vi "button commands.vi"(6 "Configuration":T1, 8 "Motion":T2, 9 "Y Steps":dbl, 10 "mapped gp buttons":T3, 11 "X Steps":dbl) -> (0 "Y distance":dbl, 1 "Choose Button":bool, 3 "X distance":dbl)   [LabVIEW 2012]
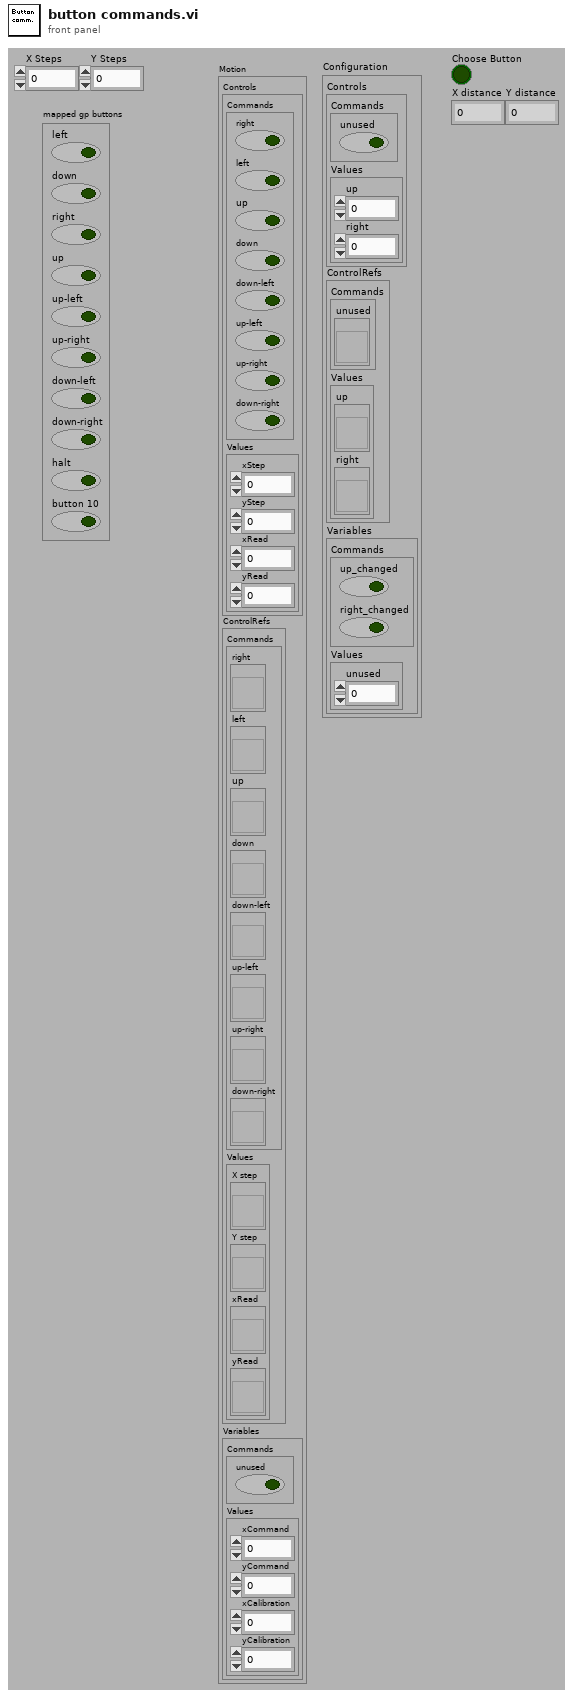
[diagram p1: front panel]
types:
  T1 = cluster{"Controls":cluster{"Commands":cluster{"unused":bool}, "Values":cluster{"up":u16, "right":u16}}, "ControlRefs":cluster{"Commands":cluster{"unused":refnum<vi>}, "Values":cluster{"up":refnum<vi>, "right":refnum<vi>}}, "Variables":cluster{"Commands":cluster{"up_changed":bool, "right_changed":bool}, "Values":cluster{"unused":i32}}}
  T2 = cluster{"Controls":cluster{"Commands":cluster{"right":bool, "left":bool, "up":bool, "down":bool, "down-left":bool, "up-left":bool, "up-right":bool, "down-right":bool}, "Values":cluster{"xStep":dbl, "yStep":dbl, "xRead":dbl, "yRead":dbl}}, "ControlRefs":cluster{"Commands":cluster{"right":refnum<vi>, "left":refnum<vi>, "up":refnum<vi>, "down":refnum<vi>, "down-left":refnum<vi>, "up-left":refnum<vi>, "up-right":refnum<vi>, "down-right":refnum<vi>}, "Values":cluster{"X step":refnum<vi>, "Y step":refnum<vi>, "xRead":refnum<vi>, "yRead":refnum<vi>}}, "Variables":cluster{"Commands":cluster{"unused":bool}, "Values":cluster{"xCommand":dbl, "yCommand":dbl, "xCalibration":dbl, "yCalibration":dbl}}}
  T3 = cluster{"left":bool, "down":bool, "right":bool, "up":bool, "up-left":bool, "up-right":bool, "down-left":bool, "down-right":bool, "halt":bool, "button 10":bool}
  T4 = cluster{"xf":bool, "xr":bool, "yf":bool, "yr":bool, "yr xr":bool, "yf xr":bool, "yf xf":bool, "yr xf":bool}
  T5 = cluster{"up":bool, "down":bool, "left":bool, "right":bool}
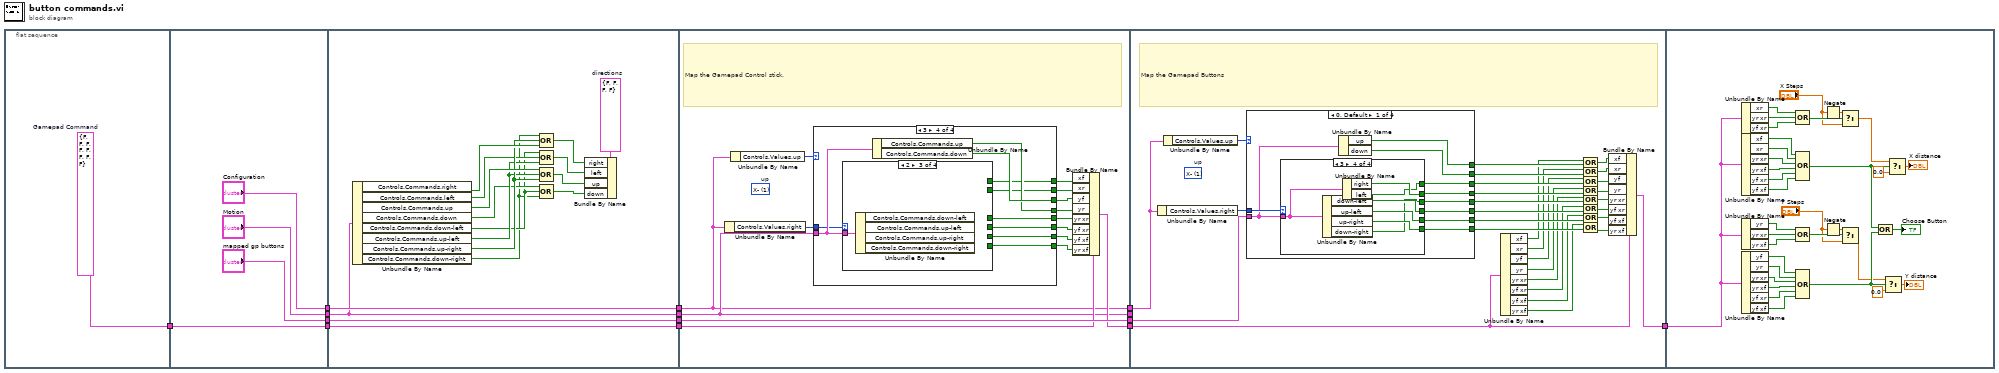
[diagram p0: block diagram]
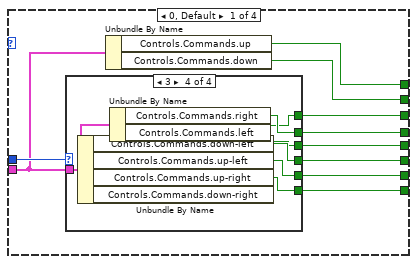
[diagram p2: hidden frame]
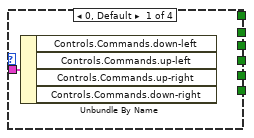
[diagram p3: hidden frame]
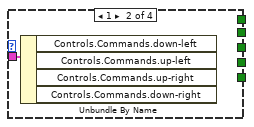
[diagram p4: hidden frame]
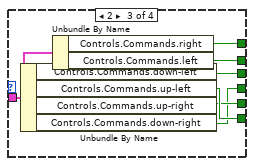
[diagram p5: hidden frame]
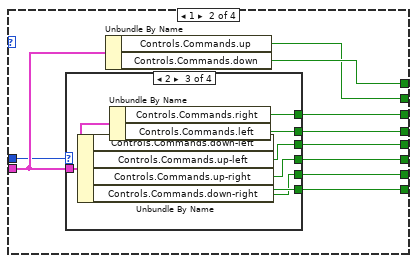
[diagram p6: hidden frame]
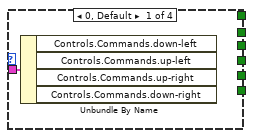
[diagram p7: hidden frame]
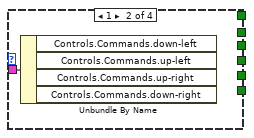
[diagram p8: hidden frame]
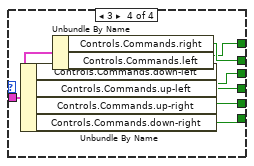
[diagram p9: hidden frame]
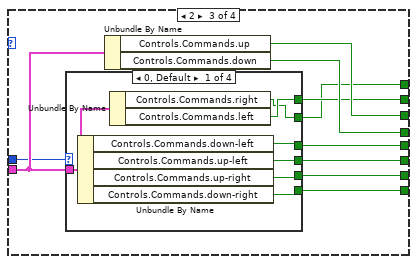
[diagram p10: hidden frame]
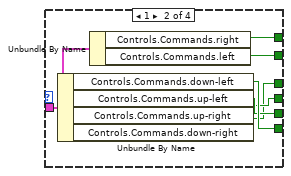
[diagram p11: hidden frame]
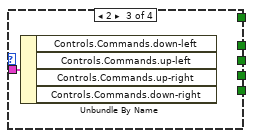
[diagram p12: hidden frame]
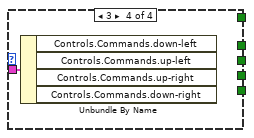
[diagram p13: hidden frame]
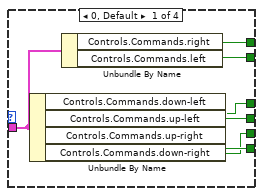
[diagram p14: hidden frame]
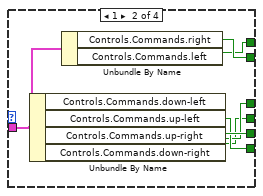
[diagram p15: hidden frame]
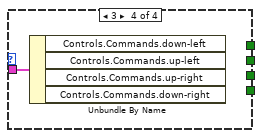
[diagram p16: hidden frame]
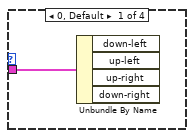
[diagram p17: hidden frame]
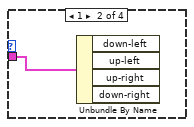
[diagram p18: hidden frame]
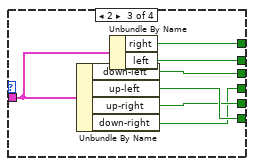
[diagram p19: hidden frame]
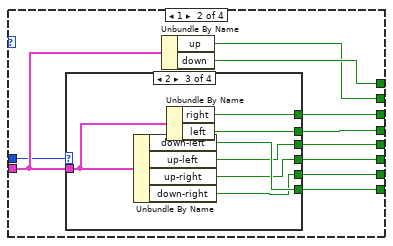
[diagram p20: hidden frame]
diagram:
  n1 = flat-sequence {
    tunnel: [w15] -> w10
    tunnel: ["mapped gp buttons"] -> w9
    tunnel: [w17] -> w8
    tunnel: ["Motion"] -> w7
    tunnel: w10 -> [w17]
    tunnel: ["Configuration"] -> w6
    tunnel: w9 -> [w36]
    tunnel: [w36] -> w5
    tunnel: w8 -> [w35]
    tunnel: [w35] -> w4
    tunnel: w7 -> [w33]
    tunnel: [w33] -> w3
    tunnel: w6 -> [w34]
    tunnel: [w34] -> w2
    tunnel: [w51] -> w13
    tunnel: [w49] -> w12
    tunnel: [w46] -> w11
    tunnel: w2 -> [w37]
    tunnel: w3 -> [w46]
    tunnel: w4 -> [w50]
    tunnel: w5 -> [w51]
    tunnel: [w37] -> w1
    tunnel: w13 -> [w180]
    tunnel: w12 -> [w164]
    tunnel: [w181] -> w14
    tunnel: w11 -> [_]
    tunnel: w1 -> [w182]
    tunnel: w14 -> [w290]
    frame #0 {
      w15 = T4 {"xf"=FALSE, "xr"=FALSE, "yf"=FALSE, "yr"=FALSE, "yr xr"=FALSE, "yf xr"=FALSE, "yf xf"=FALSE, "yr xf"=FALSE}  # Gamepad Command
    }
    frame #1 {
    }
    frame #2 {
      w32 = T5 {"up"=FALSE, "down"=FALSE, "left"=FALSE, "right"=FALSE}  # directions
      n2 = Unbundle By Name(w33) -> ("Controls.Commands.right"=w30:bool, "Controls.Commands.left"=w28:bool, "Controls.Commands.up"=w31:bool, "Controls.Commands.down"=w26:bool, "Controls.Commands.down-left"=w25:bool, "Controls.Commands.up-left"=w27:bool, "Controls.Commands.up-right"=w29:bool, "Controls.Commands.down-right"=w24:bool)
      n3 = Compound Arithmetic op=OR(w24, w29, w30) -> (w23:bool)
      n4 = Compound Arithmetic op=OR(w25, w28, w27) -> (w22:bool)
      n5 = Compound Arithmetic op=OR(w31, w27, w29) -> (w21:bool)
      n6 = Compound Arithmetic op=OR(w26, w25, w24) -> (w20:bool)
      n7 = Bundle By Name(cluster=w32, "right"=w23, "left"=w22, "up"=w21, "down"=w20) -> ()  [unwired: 1 out]
    }
    frame #3 {
      (unwired) u16 1 items=["X+", "X-", "Y+", "Y-"]  # up
      # "Map the Gamepad Control stick."
      n8 = Unbundle By Name(w37) -> ("Controls.Values.right"=w45:u16)
      n9 = Unbundle By Name(w37) -> ("Controls.Values.up"=w48:u16)
      n10 = case shown="3" w48 {
        tunnel: [w61 w81 w104 w130] -> w47
        tunnel: w46 -> [w54 w87 w113 w139]
        tunnel: w45 -> [w60 w86 w112 w138]
        tunnel: [w59 w80 w105 w131] -> w44
        tunnel: [w58 w85 w111 w137] -> w43
        tunnel: [w57 w84 w110 w136] -> w42
        tunnel: [w56 w83 w109 w135] -> w41
        tunnel: [w55 w82 w108 w134] -> w40
        tunnel: [w53 w78 w107 w133] -> w39
        tunnel: [w52 w79 w106 w132] -> w38
        frame 0, Default {
          n11 = case shown="3" w60 {
            tunnel: w54 -> [w62 w63 w66 w73]
            tunnel: [_ _ w70 w74] -> w58
            tunnel: [_ _ w69 w75] -> w57
            tunnel: [_ _ w68 w76] -> w56
            tunnel: [_ _ w67 w77] -> w55
            tunnel: [_ _ w65 w71] -> w53
            tunnel: [_ _ w64 w72] -> w52
            frame 0, Default {
              n12 = Unbundle By Name(w62) -> ()  [unwired: 4 out]
            }
            frame 1 {
              n13 = Unbundle By Name(w63) -> ()  [unwired: 4 out]
            }
            frame 2 {
              n14 = Unbundle By Name(w66) -> ("Controls.Commands.down-left"=w70:bool, "Controls.Commands.up-left"=w69:bool, "Controls.Commands.up-right"=w68:bool, "Controls.Commands.down-right"=w67:bool)
              n15 = Unbundle By Name(w66) -> ("Controls.Commands.right"=w65:bool, "Controls.Commands.left"=w64:bool)
            }
            frame 3 {
              n16 = Unbundle By Name(w73) -> ("Controls.Commands.down-left"=w77:bool, "Controls.Commands.up-left"=w76:bool, "Controls.Commands.up-right"=w75:bool, "Controls.Commands.down-right"=w74:bool)
              n17 = Unbundle By Name(w73) -> ("Controls.Commands.right"=w72:bool, "Controls.Commands.left"=w71:bool)
            }
          }
          n18 = Unbundle By Name(w54) -> ("Controls.Commands.up"=w61:bool, "Controls.Commands.down"=w59:bool)
        }
        frame 1 {
          n19 = case shown="2" w86 {
            tunnel: w87 -> [w88 w89 w92 w99]
            tunnel: [_ _ w95 w101] -> w85
            tunnel: [_ _ w96 w100] -> w84
            tunnel: [_ _ w93 w103] -> w83
            tunnel: [_ _ w94 w102] -> w82
            tunnel: [_ _ w90 w98] -> w79
            tunnel: [_ _ w91 w97] -> w78
            frame 0, Default {
              n20 = Unbundle By Name(w88) -> ()  [unwired: 4 out]
            }
            frame 1 {
              n21 = Unbundle By Name(w89) -> ()  [unwired: 4 out]
            }
            frame 2 {
              n22 = Unbundle By Name(w92) -> ("Controls.Commands.down-left"=w96:bool, "Controls.Commands.up-left"=w95:bool, "Controls.Commands.up-right"=w94:bool, "Controls.Commands.down-right"=w93:bool)
              n23 = Unbundle By Name(w92) -> ("Controls.Commands.right"=w91:bool, "Controls.Commands.left"=w90:bool)
            }
            frame 3 {
              n24 = Unbundle By Name(w99) -> ("Controls.Commands.down-left"=w103:bool, "Controls.Commands.up-left"=w102:bool, "Controls.Commands.up-right"=w101:bool, "Controls.Commands.down-right"=w100:bool)
              n25 = Unbundle By Name(w99) -> ("Controls.Commands.right"=w98:bool, "Controls.Commands.left"=w97:bool)
            }
          }
          n26 = Unbundle By Name(w87) -> ("Controls.Commands.up"=w80:bool, "Controls.Commands.down"=w81:bool)
        }
        frame 2 {
          n27 = case shown="0, Default" w112 {
            tunnel: w113 -> [w116 w123 w128 w129]
            tunnel: [w120 w124 _ _] -> w111
            tunnel: [w117 w127 _ _] -> w110
            tunnel: [w118 w126 _ _] -> w109
            tunnel: [w119 w125 _ _] -> w108
            tunnel: [w115 w122 _ _] -> w105
            tunnel: [w114 w121 _ _] -> w104
            frame 0, Default {
              n28 = Unbundle By Name(w116) -> ("Controls.Commands.down-left"=w120:bool, "Controls.Commands.up-left"=w119:bool, "Controls.Commands.up-right"=w118:bool, "Controls.Commands.down-right"=w117:bool)
              n29 = Unbundle By Name(w116) -> ("Controls.Commands.right"=w114:bool, "Controls.Commands.left"=w115:bool)
            }
            frame 1 {
              n30 = Unbundle By Name(w123) -> ("Controls.Commands.down-left"=w127:bool, "Controls.Commands.up-left"=w126:bool, "Controls.Commands.up-right"=w125:bool, "Controls.Commands.down-right"=w124:bool)
              n31 = Unbundle By Name(w123) -> ("Controls.Commands.right"=w122:bool, "Controls.Commands.left"=w121:bool)
            }
            frame 2 {
              n32 = Unbundle By Name(w128) -> ()  [unwired: 4 out]
            }
            frame 3 {
              n33 = Unbundle By Name(w129) -> ()  [unwired: 4 out]
            }
          }
          n34 = Unbundle By Name(w113) -> ("Controls.Commands.up"=w107:bool, "Controls.Commands.down"=w106:bool)
        }
        frame 3 {
          n35 = case shown="2" w138 {
            tunnel: w139 -> [w142 w149 w154 w155]
            tunnel: [w145 w151 _ _] -> w137
            tunnel: [w144 w152 _ _] -> w136
            tunnel: [w143 w153 _ _] -> w135
            tunnel: [w146 w150 _ _] -> w134
            tunnel: [w140 w148 _ _] -> w131
            tunnel: [w141 w147 _ _] -> w130
            frame 0, Default {
              n36 = Unbundle By Name(w142) -> ("Controls.Commands.down-left"=w146:bool, "Controls.Commands.up-left"=w145:bool, "Controls.Commands.up-right"=w144:bool, "Controls.Commands.down-right"=w143:bool)
              n37 = Unbundle By Name(w142) -> ("Controls.Commands.right"=w141:bool, "Controls.Commands.left"=w140:bool)
            }
            frame 1 {
              n38 = Unbundle By Name(w149) -> ("Controls.Commands.down-left"=w153:bool, "Controls.Commands.up-left"=w152:bool, "Controls.Commands.up-right"=w151:bool, "Controls.Commands.down-right"=w150:bool)
              n39 = Unbundle By Name(w149) -> ("Controls.Commands.right"=w148:bool, "Controls.Commands.left"=w147:bool)
            }
            frame 2 {
              n40 = Unbundle By Name(w154) -> ()  [unwired: 4 out]
            }
            frame 3 {
              n41 = Unbundle By Name(w155) -> ()  [unwired: 4 out]
            }
          }
          n42 = Unbundle By Name(w139) -> ("Controls.Commands.up"=w132:bool, "Controls.Commands.down"=w133:bool)
        }
      }
      n43 = Bundle By Name(cluster=w50, "xf"=w47, "xr"=w44, "yf"=w39, "yr"=w38, "yr xr"=w43, "yf xr"=w40, "yf xf"=w41, "yr xf"=w42) -> (w49:T4)
    }
    frame #4 {
      (unwired) u16 1 items=["X+", "X-", "Y+", "Y-"]  # up
      # "Map the Gamepad Buttons"
      n44 = Unbundle By Name(w182) -> ("Controls.Values.right"=w185:u16)
      n45 = Unbundle By Name(w182) -> ("Controls.Values.up"=w183:u16)
      n46 = case shown="0, Default" w183 {
        tunnel: [w195 w215 w238 w264] -> w184
        tunnel: w180 -> [w188 w221 w247 w273]
        tunnel: w185 -> [w194 w220 w246 w272]
        tunnel: [w193 w214 w239 w265] -> w178
        tunnel: [w192 w219 w245 w271] -> w175
        tunnel: [w191 w218 w244 w270] -> w172
        tunnel: [w190 w217 w243 w269] -> w173
        tunnel: [w189 w216 w242 w268] -> w174
        tunnel: [w187 w212 w241 w267] -> w177
        tunnel: [w186 w213 w240 w266] -> w176
        frame 0, Default {
          n47 = case shown="3" w194 {
            tunnel: w188 -> [w196 w197 w200 w207]
            tunnel: [_ _ w204 w208] -> w192
            tunnel: [_ _ w203 w209] -> w191
            tunnel: [_ _ w202 w210] -> w190
            tunnel: [_ _ w201 w211] -> w189
            tunnel: [_ _ w199 w205] -> w187
            tunnel: [_ _ w198 w206] -> w186
            frame 0, Default {
              n48 = Unbundle By Name(w196) -> ()  [unwired: 4 out]
            }
            frame 1 {
              n49 = Unbundle By Name(w197) -> ()  [unwired: 4 out]
            }
            frame 2 {
              n50 = Unbundle By Name(w200) -> ("down-left"=w204:bool, "up-left"=w203:bool, "up-right"=w202:bool, "down-right"=w201:bool)
              n51 = Unbundle By Name(w200) -> ("right"=w199:bool, "left"=w198:bool)
            }
            frame 3 {
              n52 = Unbundle By Name(w207) -> ("down-left"=w211:bool, "up-left"=w210:bool, "up-right"=w209:bool, "down-right"=w208:bool)
              n53 = Unbundle By Name(w207) -> ("right"=w206:bool, "left"=w205:bool)
            }
          }
          n54 = Unbundle By Name(w188) -> ("up"=w195:bool, "down"=w193:bool)
        }
        frame 1 {
          n55 = case shown="2" w220 {
            tunnel: w221 -> [w222 w223 w226 w233]
            tunnel: [_ _ w229 w235] -> w219
            tunnel: [_ _ w230 w234] -> w218
            tunnel: [_ _ w227 w237] -> w217
            tunnel: [_ _ w228 w236] -> w216
            tunnel: [_ _ w224 w232] -> w213
            tunnel: [_ _ w225 w231] -> w212
            frame 0, Default {
              n56 = Unbundle By Name(w222) -> ()  [unwired: 4 out]
            }
            frame 1 {
              n57 = Unbundle By Name(w223) -> ()  [unwired: 4 out]
            }
            frame 2 {
              n58 = Unbundle By Name(w226) -> ("down-left"=w230:bool, "up-left"=w229:bool, "up-right"=w228:bool, "down-right"=w227:bool)
              n59 = Unbundle By Name(w226) -> ("right"=w225:bool, "left"=w224:bool)
            }
            frame 3 {
              n60 = Unbundle By Name(w233) -> ("down-left"=w237:bool, "up-left"=w236:bool, "up-right"=w235:bool, "down-right"=w234:bool)
              n61 = Unbundle By Name(w233) -> ("right"=w232:bool, "left"=w231:bool)
            }
          }
          n62 = Unbundle By Name(w221) -> ("up"=w214:bool, "down"=w215:bool)
        }
        frame 2 {
          n63 = case shown="0, Default" w246 {
            tunnel: w247 -> [w250 w257 w262 w263]
            tunnel: [w254 w258 _ _] -> w245
            tunnel: [w251 w261 _ _] -> w244
            tunnel: [w252 w260 _ _] -> w243
            tunnel: [w253 w259 _ _] -> w242
            tunnel: [w249 w256 _ _] -> w239
            tunnel: [w248 w255 _ _] -> w238
            frame 0, Default {
              n64 = Unbundle By Name(w250) -> ("down-left"=w254:bool, "up-left"=w253:bool, "up-right"=w252:bool, "down-right"=w251:bool)
              n65 = Unbundle By Name(w250) -> ("right"=w248:bool, "left"=w249:bool)
            }
            frame 1 {
              n66 = Unbundle By Name(w257) -> ("down-left"=w261:bool, "up-left"=w260:bool, "up-right"=w259:bool, "down-right"=w258:bool)
              n67 = Unbundle By Name(w257) -> ("right"=w256:bool, "left"=w255:bool)
            }
            frame 2 {
              n68 = Unbundle By Name(w262) -> ()  [unwired: 4 out]
            }
            frame 3 {
              n69 = Unbundle By Name(w263) -> ()  [unwired: 4 out]
            }
          }
          n70 = Unbundle By Name(w247) -> ("up"=w241:bool, "down"=w240:bool)
        }
        frame 3 {
          n71 = case shown="2" w272 {
            tunnel: w273 -> [w276 w283 w288 w289]
            tunnel: [w279 w285 _ _] -> w271
            tunnel: [w278 w286 _ _] -> w270
            tunnel: [w277 w287 _ _] -> w269
            tunnel: [w280 w284 _ _] -> w268
            tunnel: [w274 w282 _ _] -> w265
            tunnel: [w275 w281 _ _] -> w264
            frame 0, Default {
              n72 = Unbundle By Name(w276) -> ("down-left"=w280:bool, "up-left"=w279:bool, "up-right"=w278:bool, "down-right"=w277:bool)
              n73 = Unbundle By Name(w276) -> ("right"=w275:bool, "left"=w274:bool)
            }
            frame 1 {
              n74 = Unbundle By Name(w283) -> ("down-left"=w287:bool, "up-left"=w286:bool, "up-right"=w285:bool, "down-right"=w284:bool)
              n75 = Unbundle By Name(w283) -> ("right"=w282:bool, "left"=w281:bool)
            }
            frame 2 {
              n76 = Unbundle By Name(w288) -> ()  [unwired: 4 out]
            }
            frame 3 {
              n77 = Unbundle By Name(w289) -> ()  [unwired: 4 out]
            }
          }
          n78 = Unbundle By Name(w273) -> ("up"=w266:bool, "down"=w267:bool)
        }
      }
      n79 = Unbundle By Name(w164) -> ("xf"=w163:bool, "xr"=w162:bool, "yf"=w161:bool, "yr"=w160:bool, "yr xr"=w159:bool, "yf xr"=w158:bool, "yf xf"=w157:bool, "yr xf"=w156:bool)
      n80 = Compound Arithmetic op=OR(w163, w184) -> (w179:bool)
      n81 = Compound Arithmetic op=OR(w162, w178) -> (w171:bool)
      n82 = Compound Arithmetic op=OR(w161, w177) -> (w170:bool)
      n83 = Compound Arithmetic op=OR(w160, w176) -> (w169:bool)
      n84 = Compound Arithmetic op=OR(w159, w175) -> (w168:bool)
      n85 = Compound Arithmetic op=OR(w158, w174) -> (w167:bool)
      n86 = Compound Arithmetic op=OR(w157, w173) -> (w166:bool)
      n87 = Compound Arithmetic op=OR(w156, w172) -> (w165:bool)
      n88 = Bundle By Name(cluster=w164, "xf"=w179, "xr"=w171, "yf"=w170, "yr"=w169, "yr xr"=w168, "yf xr"=w167, "yf xf"=w166, "yr xf"=w165) -> (w181:T4)
    }
    frame #5 {
      n89 = Unbundle By Name(w290) -> ("xr"=w295:bool, "yr xr"=w296:bool, "yf xr"=w297:bool)
      n90 = Unbundle By Name(w290) -> ("xf"=w304:bool, "xr"=w305:bool, "yr xr"=w306:bool, "yr xf"=w307:bool, "yf xr"=w308:bool, "yf xf"=w309:bool)
      n91 = Unbundle By Name(w290) -> ("yr"=w313:bool, "yr xr"=w312:bool, "yr xf"=w311:bool)
      n92 = Unbundle By Name(w290) -> ("yf"=w298:bool, "yr"=w299:bool, "yr xr"=w300:bool, "yr xf"=w301:bool, "yf xr"=w302:bool, "yf xf"=w303:bool)
      n93 = Compound Arithmetic op=OR(w295, w296, w297) -> (w310:bool)
      n94 = Compound Arithmetic op=OR(w304, w305, w306, w307, w308, w309) -> (w321:bool)
      n95 = Compound Arithmetic op=OR(w313, w312, w311) -> (w314:bool)
      n96 = Compound Arithmetic op=OR(w298, w299, w300, w301, w302, w303) -> (w322:bool)
      n97 = Negate(x="X Steps") -> (-x=w291:dbl)
      n98 = Negate(x="Y Steps") -> (-x=w293:dbl)
      n99 = Select(t=w291, s=w310, f="X Steps") -> (s? t:f=w317:dbl)
      n100 = Select(t=w293, s=w314, f="Y Steps") -> (s? t:f=w315:dbl)
      n101 = Compound Arithmetic op=OR(w321, w322) -> (→"Choose Button":bool)
      n102 = Select(t=w315, s=w322, f=0.0) -> (s? t:f=→"Y distance":dbl)
      n103 = Select(t=w317, s=w321, f=0.0) -> (s? t:f=→"X distance":dbl)
    }
  }
